vi "Get_requested_rows_from_files.vi"(3 "Last File":bool, 4 "First file":bool, 5 "Filename":path, 6 "Selected Rows":i32[](array[numeric])) -> ()   [LabVIEW 2014]
uses:
  Globals/Constants_global.vi
panel:
  out "Ch names Out":string[](array[string])
  out "Channel Values Out":string[][](array[string])
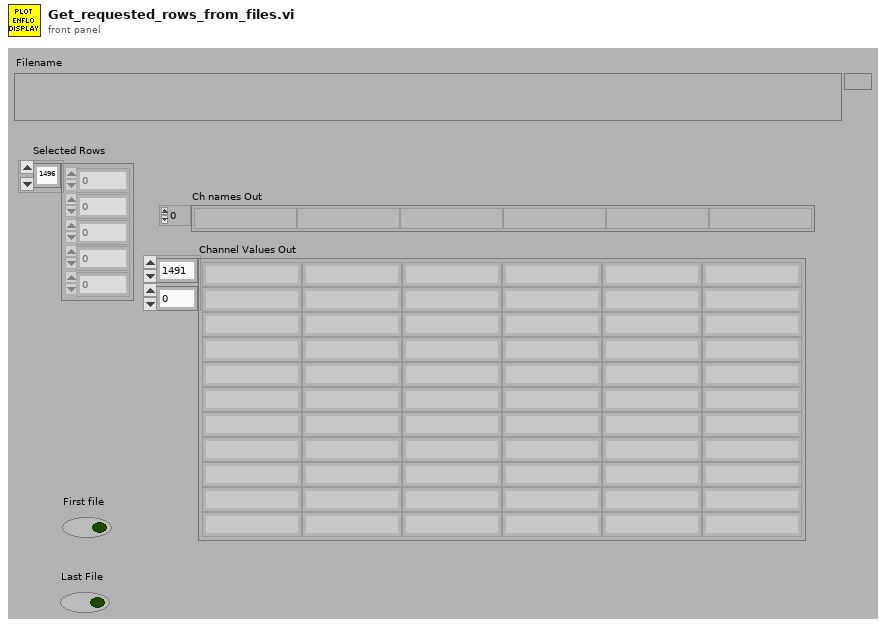
[diagram p1: front panel]
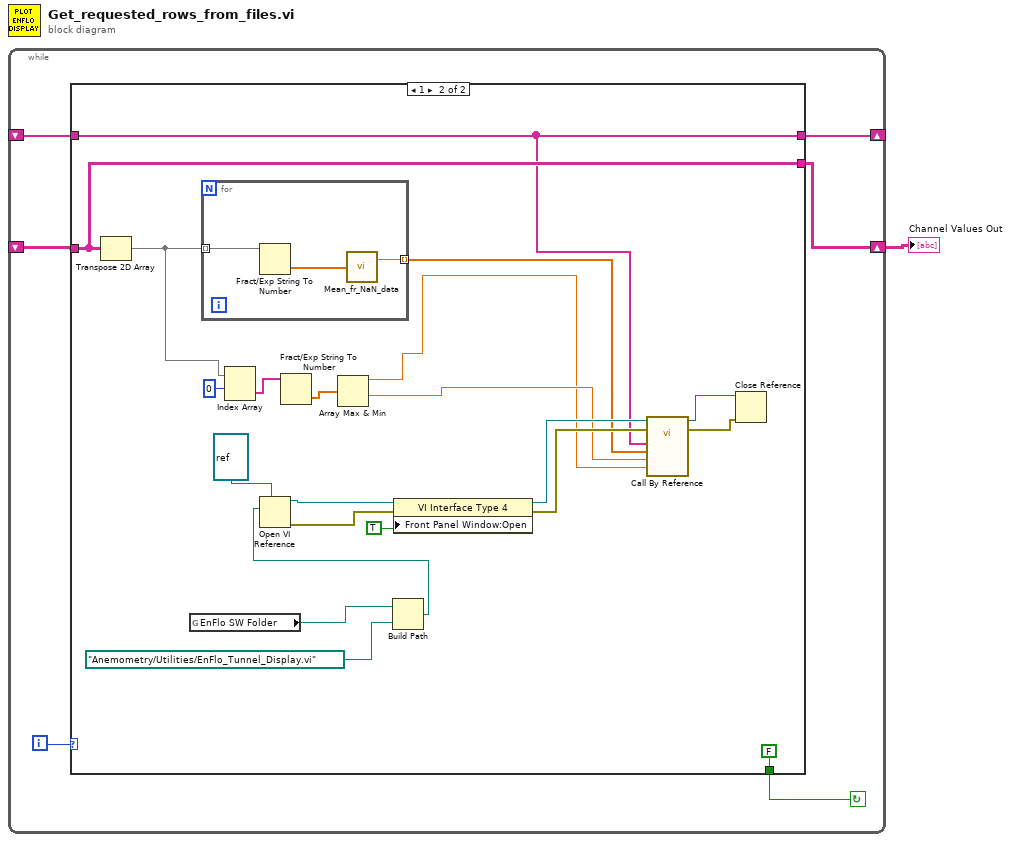
[diagram p0: block diagram]
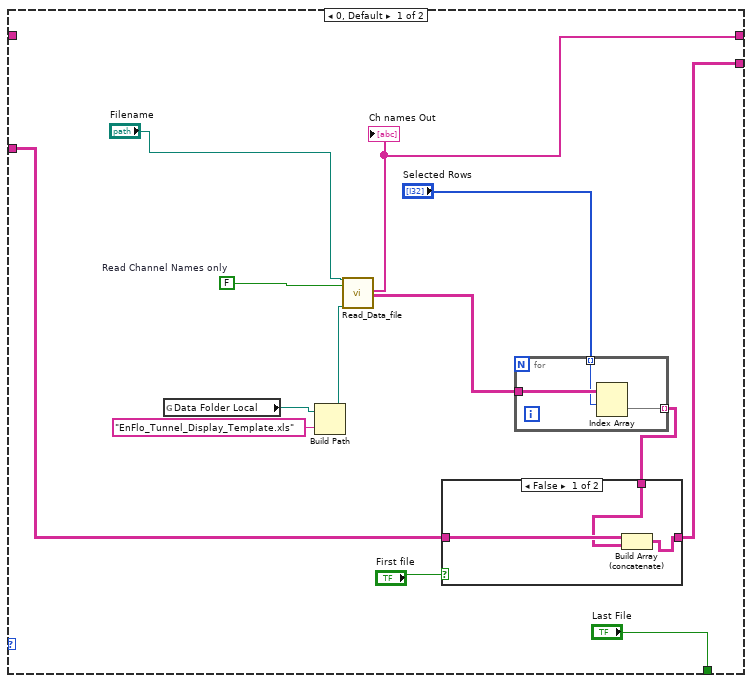
[diagram p2: hidden frame]
diagram:
  n1 = while {
    shift-right: [w6] -> w1
    shift-left: _ -> [w7]
    shift-right: [w4] -> _
    shift-left: _ -> [w3]
    i -> [w2]
    stop <- w5 continue-if-true
    n2 = case shown="1" w2 {
      tunnel: [w12 w48] -> w6
      tunnel: w7 -> [w11 w48]
      tunnel: ["Last File" FALSE ("Last File")] -> w5
      tunnel: [w9 w31] -> w4
      tunnel: w3 -> [_ w31]
      frame 0, Default {
        w16 = FALSE  # Read Channel Names only
        n3 = global read "Constants_global.vi" "Data Folder Local"() -> (w18:path)
        n4 = Build Path(base path=w18, name or relative path="EnFlo_Tunnel_Display_Template.xls") -> (appended path=w19:path)
        n5 = call "Read_Data_file.vi"("Results file"="Filename", "Read Channel Names only"=w16, "Template File"=w19) -> ("Ch names Out"=w9:string[], "Channel Values Out"=w20:string[][])  [unwired: 2 in, 13 out]
        "Ch names Out" <- w9
        n6 = for {
          tunnel: w20 -> [w27]
          tunnel: "Selected Rows" -> [w26] mode=indexing
          tunnel: [w25] -> w13 mode=indexing
          n7 = Index Array(array=w27, index (row)=w26) -> (element=w25:string[])  [unwired: 1 in]
        }
        n8 = case shown="False" "First file" {
          tunnel: [w21 w24] -> w12
          tunnel: w13 -> [w22 w24]
          tunnel: w11 -> [w23 _]
          frame False {
            n9 = Build Array (concatenate)(w23, w22) -> (w21:string[][])
          }
          frame True {
          }
        }
      }
      frame 1 {
        n10 = Transpose 2D Array(2D array=w48) -> (transposed array=w46:string[][])
        n11 = global read "Constants_global.vi" "EnFlo SW Folder"() -> (w42:path)
        n12 = for {
          tunnel: w46 -> [w51] mode=indexing
          tunnel: [w50] -> w30 mode=indexing
          n13 = Fract/Exp String To Number(string=w51) -> (number=w49:dbl[])  [unwired: 3 in, 1 out]
          n14 = call "Mean_fr_NaN_data.vi"("Data"=w49) -> ("Mean value"=w50:dbl)  [unwired: 1 out]
        }
        n15 = Index Array(array=w46, index (row)=0) -> (element=w44:string[])  [unwired: 1 in]
        n16 = Fract/Exp String To Number(string=w44) -> (number=w43:dbl[])  [unwired: 3 in, 1 out]
        n17 = Array Max & Min(array=w43) -> (max value=w28:dbl, min value=w29:dbl)  [unwired: 2 out]
        n18 = Build Path(base path=w42, name or relative path=path "Anemometry/Utilities/EnFlo_Tunnel_Display.vi") -> (appended path=w38:path)
        n19 = Open VI Reference(type specifier VI Refnum (for type only)=refnum<vi> refnum, vi path=w38) -> (vi reference=w37:refnum<vi>, error out=w36:errorcluster)  [unwired: 1 in, 3 out]
        n20 = property class="VI Interface Type 4"(reference=w37, error in=w36, "Front Panel Window:Open"=TRUE) -> (reference out=w35:refnum<vi>, error out=w33:errorcluster)
        n21 = call-by-ref "?"(reference=w35, error in=w33, "End Time"=w28, "Start Time"=w29, "Channel Values"=w30, "Ch names"=w31) -> (reference out=w34:refnum<vi>, error out=w32:errorcluster)  [unwired: 4 in]
        n22 = Close Reference(reference=w34, error in (no error)=w32) -> ()  [unwired: 1 out]
      }
    }
  }
  "Channel Values Out" <- w1
